vi "Read Loc String.vi"(10 "Error In":errorcluster, 11 "Loc String .NET Ref":refnum<k24>) -> (2 "Error Out":errorcluster, 3 "English":string, 5 "Localized":string)   [LabVIEW 2019, in "VeriStand Custom Device XML Parser.lvlib"]
uses:
  VeriStand Custom Device XML Parser.lvlib
  NationalInstruments.VeriStand.XMLReader
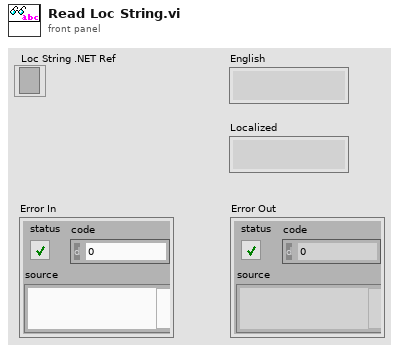
[diagram p1: front panel]
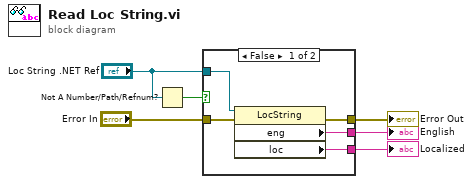
[diagram p0: block diagram]
diagram:
  n1 = Not A Number/Path/Refnum?(number/path/refnum="Loc String .NET Ref") -> (NaN/Path/Refnum?=w1:bool)
  n2 = case shown="False" w1 {
    tunnel: [w11 w12] -> w6
    tunnel: [w10 _] -> w5
    tunnel: [w9 _] -> w4
    tunnel: "Error In" -> [w8 w12]
    tunnel: "Loc String .NET Ref" -> [w7 _]
    frame False {
      n3 = property class="LocString"(reference=w7, error in=w8) -> (error out=w11:errorcluster, "eng"=w9:string, "loc"=w10:string)  [unwired: 1 out]
    }
    frame True {
    }
  }
  "Error Out" <- w6
  "Localized" <- w5
  "English" <- w4
